vi "Undo.vi"(8 "error in (no error)":errorcluster, 11 "reference in":refnum<class "CeilingFanLowCommand.lvclass">) -> (0 "error out":errorcluster, 3 "reference in":refnum<class "CeilingFanLowCommand.lvclass">)   [LabVIEW 2012, in "CeilingFanLowCommand.lvclass"]
uses:
  CeilingFanLowCommand.lvclass
  CeilingFan_class/CeilingFan.lvclass
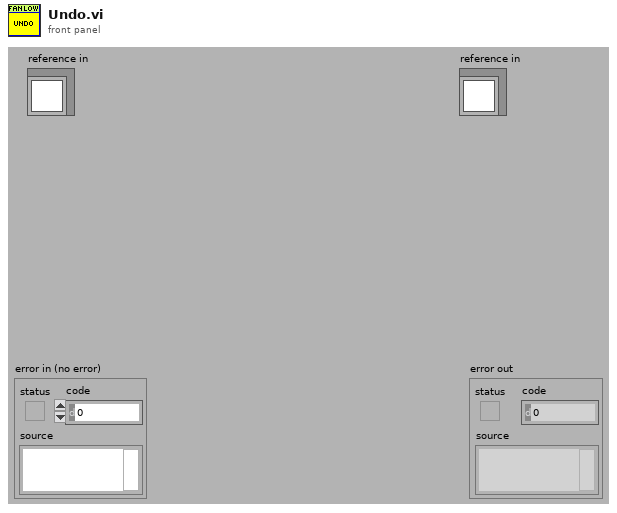
[diagram p1: front panel]
types:
  T1 = typedef "CeilingFanLowCommand.lvclass/ObjectAttributes.ctl" = cluster{"CeilingFan":refnum<class "CeilingFan.lvclass">, "PrevSpeed":i32}
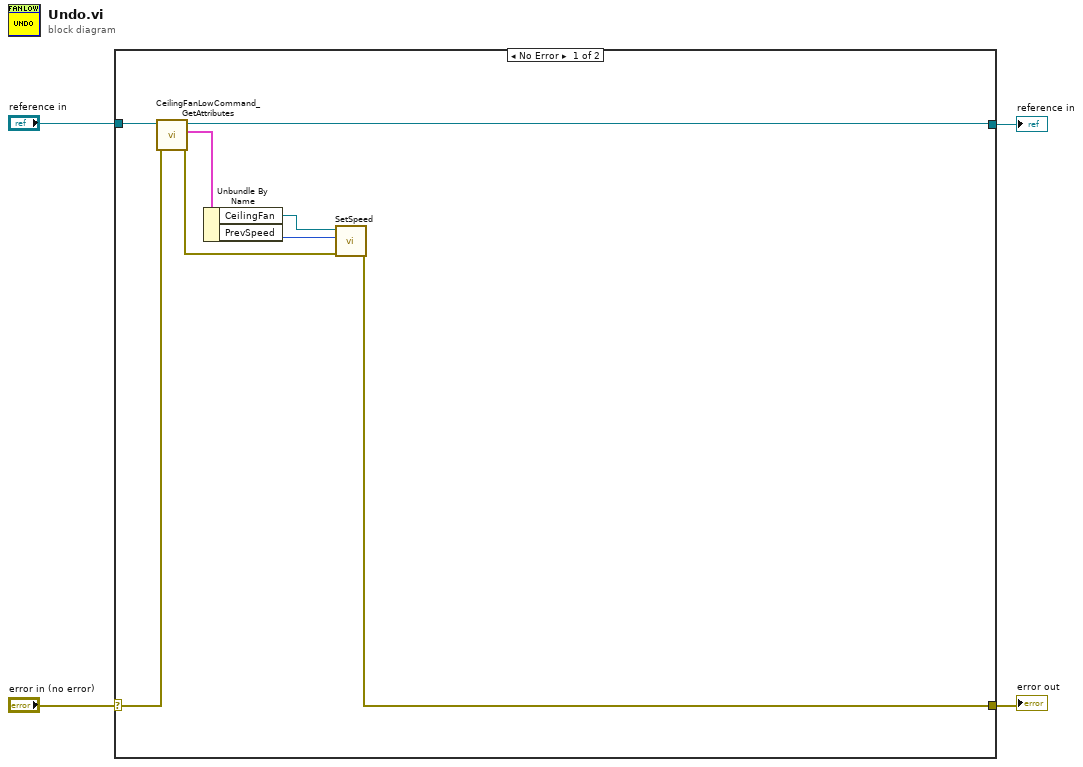
[diagram p0: block diagram]
diagram:
  n1 = case shown="No Error" "error in (no error)" {
    selector: "error in (no error)" -> [w11 w14]
    tunnel: [w5 w14] -> w3
    tunnel: [w9 w13] -> w1
    tunnel: "reference in" -> [w12 w13]
    frame No Error {
      n2 = call "CeilingFanLowCommand_GetAttributes.vi"("error in (no error)"=w11, "reference in"=w12) -> ("error out"=w6:errorcluster, "Data"=w10:T1, "reference out"=w9:refnum<class "CeilingFanLowCommand.lvclass">)  [unwired: 6 in, 1 out]
      n3 = Unbundle By Name(w10) -> ("CeilingFan"=w7:refnum<class "CeilingFan.lvclass">, "PrevSpeed"=w8:i32)
      n4 = call-dynamic "SetSpeed.vi"("error in (no error)"=w6, "Speed"=w8, "reference in"=w7) -> ("error out"=w5:errorcluster)  [unwired: 7 in, 1 out]
    }
    frame Error {
    }
  }
  "error out" <- w3
  "reference in" <- w1
